vi "Write Text.vi"(8 "error in (no error)":errorcluster, 9 "Text":string, 10 "Session In":refnum<class "Session.lvclass">, 11 "Character LCD in":refnum<class "PCF8574 I2C LCD.lvclass">) -> (0 "error out":errorcluster, 2 "Session Out":refnum<class "Session.lvclass">, 3 "Character LCD out":refnum<class "PCF8574 I2C LCD.lvclass">)   [LabVIEW 2020, in "CTI-Peripheral.lvlib" / "PCF8574 I2C LCD.lvclass"]
uses:
  PCF8574 I2C LCD.lvclass
  CTI/Session/Session.lvclass
  Mode.ctl
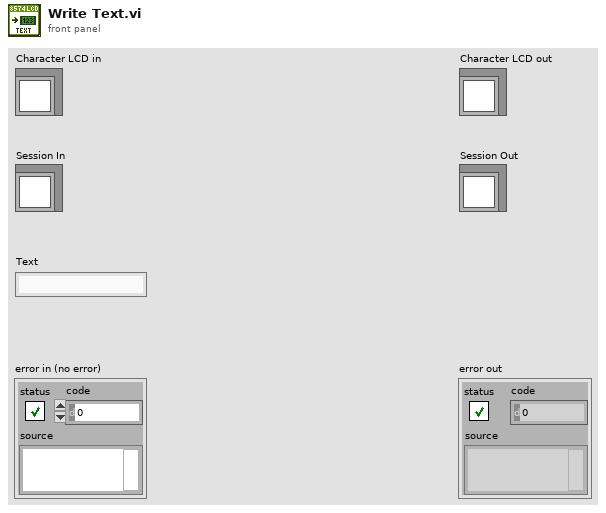
[diagram p1: front panel]
types:
  T1 = typedef "CTI-Peripheral.lvlib/PCF8574 I2C LCD.lvclass/Mode.ctl" = enum8{"Command", "Character"}
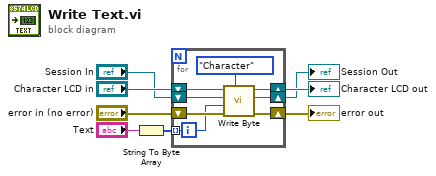
[diagram p0: block diagram]
diagram:
  n1 = String To Byte Array(string="Text") -> (unsigned byte array=w1:u8[])
  n2 = for {
    shift-right: [w15] -> w7
    shift-left: "error in (no error)" -> [w16]
    shift-right: [w13] -> w5
    shift-left: "Character LCD in" -> [w14]
    shift-right: [w10] -> w3
    shift-left: "Session In" -> [w11]
    tunnel: w1 -> [w9] mode=indexing
    n3 = call "Write Byte.vi"("Mode (Command)"=Mode."Character", "error in (no error)"=w16, "Value"=w9, "Session in"=w11, "PCF8574 I2C LCD in"=w14) -> ("error out"=w15:errorcluster, "Session out"=w10:refnum<class "Session.lvclass">, "PCF8574 I2C LCD out"=w13:refnum<class "PCF8574 I2C LCD.lvclass">)  [unwired: 4 in]
  }
  "error out" <- w7
  "Character LCD out" <- w5
  "Session Out" <- w3
